vi "Get Object Parameter - Array.vi"(8 "error in (no error)":errorcluster, 10 "Parameter Name":string, 11 "JSON Tree In (JSON Object)":variant) -> (0 "error out":errorcluster, 1 "is JSON Null?":bool, 2 "JSON Array":variant, 3 "JSON Tree Out Passthrough":variant)   [LabVIEW 2013, in "i3-json.lvlib"]
doc: "Get a named parameter from a JSON Tree Object"
uses:
  i3-json.lvlib
  JSON Types/JSON Type.ctl
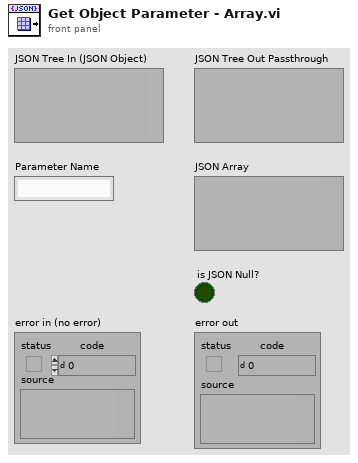
[diagram p1: front panel]
types:
  T1 = typedef "i3-json.lvlib/JSON Type.ctl" = enum8{"JSON Compatible", "JSON Array", "JSON Object", "JSON Null", "Double", "String", "Boolean", "Unknown"}
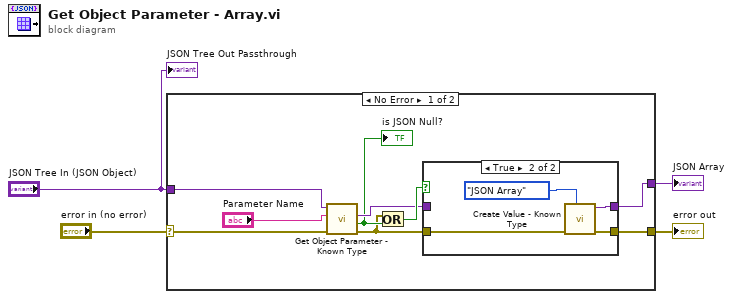
[diagram p0: block diagram]
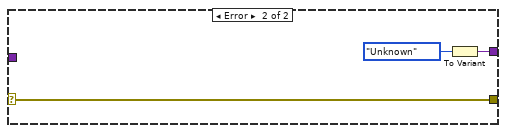
[diagram p3: hidden frame]
diagram:
  n1 = case shown="No Error" "error in (no error)" {
    selector: "error in (no error)" -> [w12 w22]
    tunnel: [w10 w22] -> w3
    tunnel: "JSON Tree In (JSON Object)" -> [w13 _]
    tunnel: [w8 w20] -> w2
    frame No Error {
      n2 = call "Get Object Parameter - Known Type.vi"("error in (no error)"=w12, "Parameter Name"="Parameter Name", "JSON Tree In (JSON Object)"=w13) -> ("error out"=w5:errorcluster, "is JSON Null?"=w7:bool, "Value"=w9:variant)  [unwired: 3 in, 3 out]
      "is JSON Null?" <- w7
      n3 = Or(x=w5, y=w7) -> (x .or. y?=w11:bool)
      n4 = case shown="True" w11 {
        tunnel: w5 -> [w14 w18]
        tunnel: [w14 w17] -> w10
        tunnel: w9 -> [w15 _]
        tunnel: [w15 w16] -> w8
        frame False {
        }
        frame True {
          n5 = call "Create Value - Known Type.vi"("JSON Type"=JSON_Type."JSON Array", "error in (no error)"=w18) -> ("error out"=w17:errorcluster, "JSON Tree"=w16:variant)  [unwired: 8 in]
        }
      }
    }
    frame Error {
      n6 = To Variant(anything=JSON_Type."Unknown" ("JSON Type")) -> (Variant=w20:variant)
    }
  }
  "error out" <- w3
  "JSON Array" <- w2
  "JSON Tree Out Passthrough" <- "JSON Tree In (JSON Object)"
